vi "Variant To Data_I4.vi"(8 "error in (no error)":errorcluster, 11 "Variant":variant) -> (0 "error out":errorcluster, 2 "OK?":bool, 3 "Data":i32[](array[numeric]))   [LabVIEW 2020, in "SECS Communication.lvlib" / "SECS-II Class.lvclass"]
uses:
  SECS-II Class.lvclass
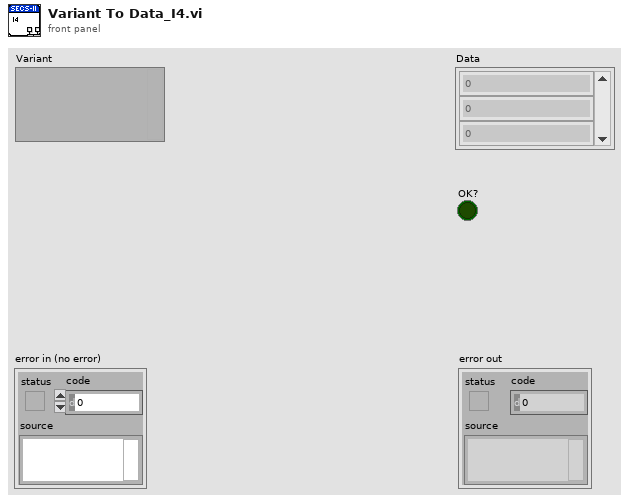
[diagram p1: front panel]
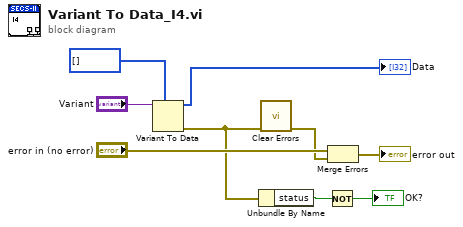
[diagram p0: block diagram]
diagram:
  n1 = Variant To Data(type=i32[] [] ("Data"), Variant="Variant") -> (data=→"Data":i32[], error out=w1:errorcluster)  [unwired: 1 in]
  n2 = Unbundle By Name(w1) -> ("status"=w3:bool)
  n3 = call <vilib>:"Clear Errors.vi"("error in (no error)"=w1) -> ("error out"=w4:errorcluster)  [unwired: 5 in, 1 out]
  n4 = Not(x=w3) -> (.not. x?=→"OK?":bool)
  n5 = Merge Errors("error in (no error)", w4) -> (→"error out":errorcluster)
